vi "LoadArray.vi"(11 "file path":path) -> (3 "data":dbl[][](array[numeric]))   [LabVIEW 2010, in "KevLib01.lvlib"]
uses:
  KevLib01.lvlib
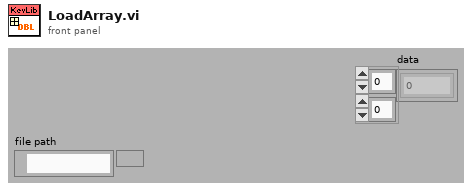
[diagram p1: front panel]
types:
  T1 = enum16{"open", "replace", "create", "open or create", "replace or create", "replace or create with confirmation"}
  T2 = enum16{"deny read/write", "deny write-only", "deny none"}
  T3 = enum16{"big-endian, network order", "native, host order", "little-endian"}
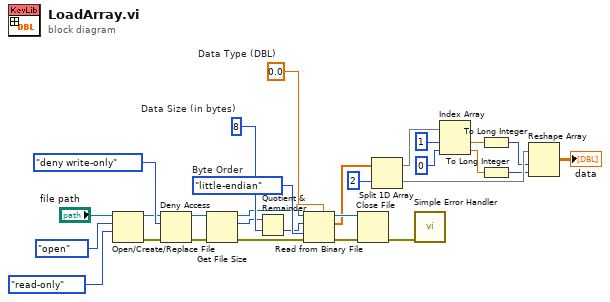
[diagram p0: block diagram]
diagram:
  w22 = T3."little-endian"  # Byte Order
  w20 = i64 8  # Data Size (in bytes)
  w19 = 0.0  # Data Type (DBL)
  n1 = Open/Create/Replace File(file path (use dialog)="file path", operation (0:open)=T1."open", access (0:read/write)=enum16{"read/write", "read-only", "write-only"}."read-only") -> (refnum out=w24:refnum<file>, error out=w23:errorcluster)  [unwired: 1 in, 3 out]
  n2 = Deny Access(4:w23, 6:T2."deny write-only" ("deny mode (0:deny read/write)"), 7:w24) -> (0:w25:errorcluster, 3:w26:refnum<file>)
  n3 = Get File Size(file=w26, error in=w25) -> (refnum out=w12:refnum<file>, size (in bytes)=w16:i64, 0:w17:errorcluster)
  n4 = Quotient & Remainder(x=w16, y=w20) -> (floor(x/y)=w21:i64)  [unwired: 1 out]
  n5 = Read from Binary File(5:w19, 8:w17, 9:w22, 10:w21, 11:w12) -> (0:w14:errorcluster, 2:w11:dbl[], 3:w13:refnum<file>)  [unwired: 2 out]
  n6 = Close File(refnum=w13, error in=w14) -> (error out=w15:errorcluster)  [unwired: 1 out]
  n7 = Split 1D Array(array=w11, index=2) -> (first subarray=w9:dbl[], second subarray=w6:dbl[])
  n8 = call <vilib>:"Simple Error Handler.vi"("error in (no error)"=w15) -> ()  [unwired: 1 in, 8 out]
  n9 = Index Array(array=w9, index #1=1 ("index"), index #2=0 ("index")) -> (element #1=w5:dbl, element #2=w4:dbl)
  n10 = To Long Integer(number=w5) -> (32bit integer=w3:i32)
  n11 = To Long Integer(number=w4) -> (32bit integer=w2:i32)
  n12 = Reshape Array(w6, w3, w2) -> (→"data":dbl[][])
